vi "Load Category Sums (TEMP).vi"(8 "error in (no error)":errorcluster, 10 "SQL Date":string, 11 "Database in":refnum<class "Database.lvclass">) -> (0 "error out":errorcluster, 2 "Bdgt Values":string[][](array[string]), 3 "Database out":refnum<class "Database.lvclass">)   [LabVIEW 2018, in "Database.lvclass"]
uses:
  Database.lvclass
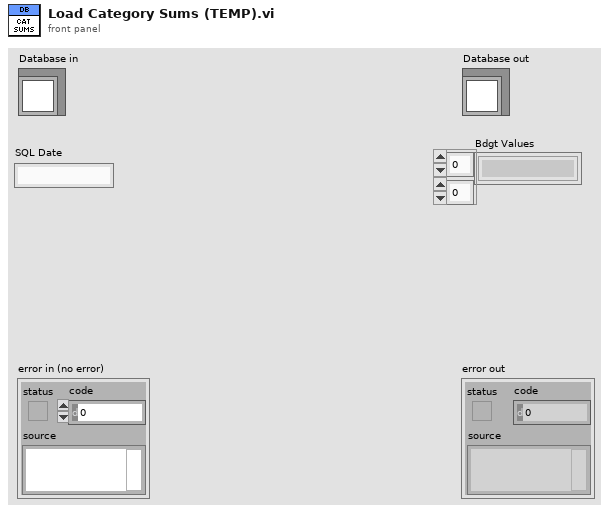
[diagram p1: front panel]
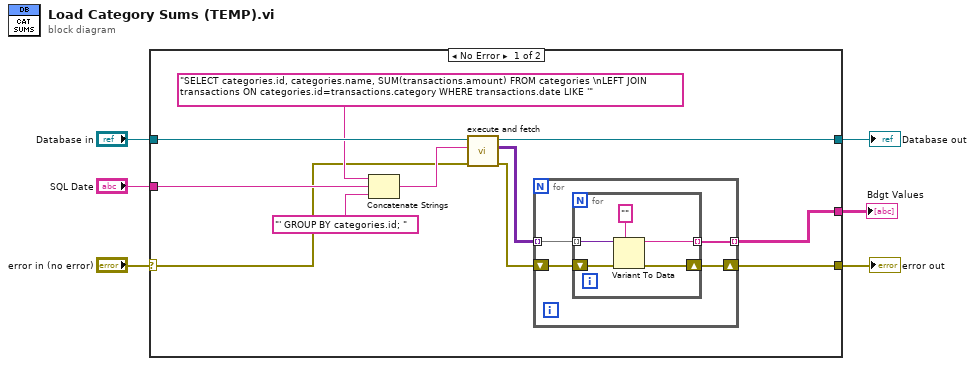
[diagram p0: block diagram]
diagram:
  n1 = case shown="No Error" "error in (no error)" {
    selector: "error in (no error)" -> [w7 w27]
    tunnel: [w14 w28] -> w6
    tunnel: "Database in" -> [w13 w28]
    tunnel: [w12 w27] -> w4
    tunnel: "SQL Date" -> [w11 _]
    tunnel: [w8 _] -> w2
    frame No Error {
      n2 = Concatenate Strings("SELECT categories.id, categories.name, SUM(transactions.amount) FROM categories \nLEFT JOIN transactions ON categories.id=transactions.category WHERE transactions.date LIKE '", w11, "' GROUP BY categories.id; ") -> (w15:string)
      n3 = call "execute and fetch.vi"("error in (no error)"=w7, "SQL query"=w15, "Database in"=w13) -> ("error out"=w16:errorcluster, "recordset data"=w17:variant[][], "Database out"=w14:refnum<class "Database.lvclass">)  [unwired: 5 in, 1 out]
      n4 = for {
        tunnel: w17 -> [w21] mode=indexing
        shift-right: [w19] -> w12
        shift-left: w16 -> [w20]
        tunnel: [w18] -> w8 mode=indexing
        n5 = for {
          tunnel: w21 -> [w26] mode=indexing
          shift-right: [w24] -> w19
          shift-left: w20 -> [w25]
          tunnel: [w22] -> w18 mode=indexing
          n6 = Variant To Data(error in=w25, type="", Variant=w26) -> (data=w22:string, error out=w24:errorcluster)
        }
      }
    }
    frame Error {
    }
  }
  "error out" <- w4
  "Database out" <- w6
  "Bdgt Values" <- w2
